vi "Compare U64 Arrays.vi"(10 "Array 2":u64[](array[numeric]), 11 "Array 1":u64[](array[numeric])) -> (2 "First Mismatch Location":u32, 3 "Equal?":bool)   [LabVIEW 2010]
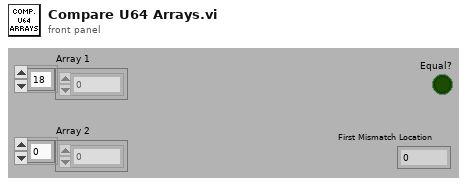
[diagram p1: front panel]
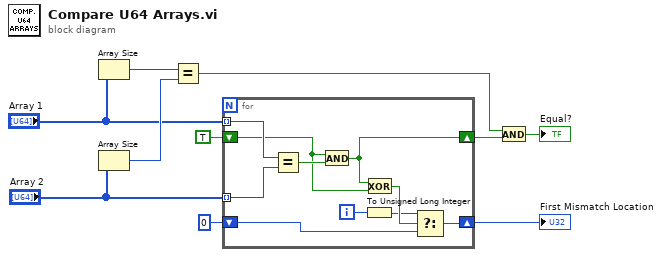
[diagram p0: block diagram]
diagram:
  n1 = Array Size(array="Array 1") -> (size(s)=w10:i32)
  n2 = Array Size(array="Array 2") -> (size(s)=w9:i32)
  n3 = Equal?(x=w10, y=w9) -> (x = y?=w1:bool)
  n4 = for {
    tunnel: "Array 1" -> [w18] mode=indexing
    tunnel: "Array 2" -> [w19] mode=indexing
    shift-right: [w16] -> w2
    shift-left: TRUE ("Equal?") -> [w17]
    shift-right: [w15] -> w4
    shift-left: u32 0 ("First Mismatch Location") -> [w14]
    i -> [w12]
    n5 = Equal?(x=w18, y=w19) -> (x = y?=w20:bool)
    n6 = And(x=w17, y=w20) -> (x .and. y?=w16:bool)
    n7 = To Unsigned Long Integer(number=w12) -> (unsigned 32bit integer=w11:u32)
    n8 = Exclusive Or(1:w17, 2:w16) -> (0:w13:bool)
    n9 = Select(t=w11, s=w13, f=w14) -> (s? t:f=w15:u32)
  }
  "First Mismatch Location" <- w4
  n10 = And(x=w1, y=w2) -> (x .and. y?=→"Equal?":bool)
